vi "setup mfc LabJack interface.vi"() -> (0 "error out":errorcluster, 3 "LabJack Tasks":T2)   [LabVIEW 2021]
uses:
  temporal odor control/LabJack Interface/LabJackSetupChannel.ctl
  temporal odor control/LabJack Interface/LabJack AOAI Channel.ctl
panel:
  in  "Output Channels":T4={"OdorFlowRate"={"LabJack"=enum."1", "LabJack Channel Number"=0.0, "Scaling"=0.1}, "Background Air Flow"={"LabJack"=enum."1", "LabJack Channel Number"=1.0, "Scaling"=0.001}, "Air Dilution"={"LabJack"=enum."2", "LabJack Channel Number"=1.0, "Scaling"=0.025}}
  out "labjack2 handle":i32
  in  "Input Channels":T5={"OdorFlowRate"={"LabJack"=enum."1", "LabJack Channel Number"=2.0, "Scaling"=10.0}, "PID outlet"={"LabJack"=enum."1", "LabJack Channel Number"=0.0, "Scaling"=1.0}, "Outlet OpticalFlowSensor"={"LabJack"=enum."2", "LabJack Channel Number"=0.0, "Scaling"=1.0}, "Background Air Flow"={"LabJack"=enum."2", "LabJack Channel Number"=1.0, "Scaling"=1000.0}, "Air Dilution"={"LabJack"=enum."2", "LabJack Channel Number"=2.0, "Scaling"=40.0}}
  out "labjack1 handle":i32
  # "sccm/V"
  # "V/sccm"
  # "V/sccm"
  # "V/sccm"
  # "white = setpoint\nyellow = flow out\ngreen = valve off\nblue = purge"
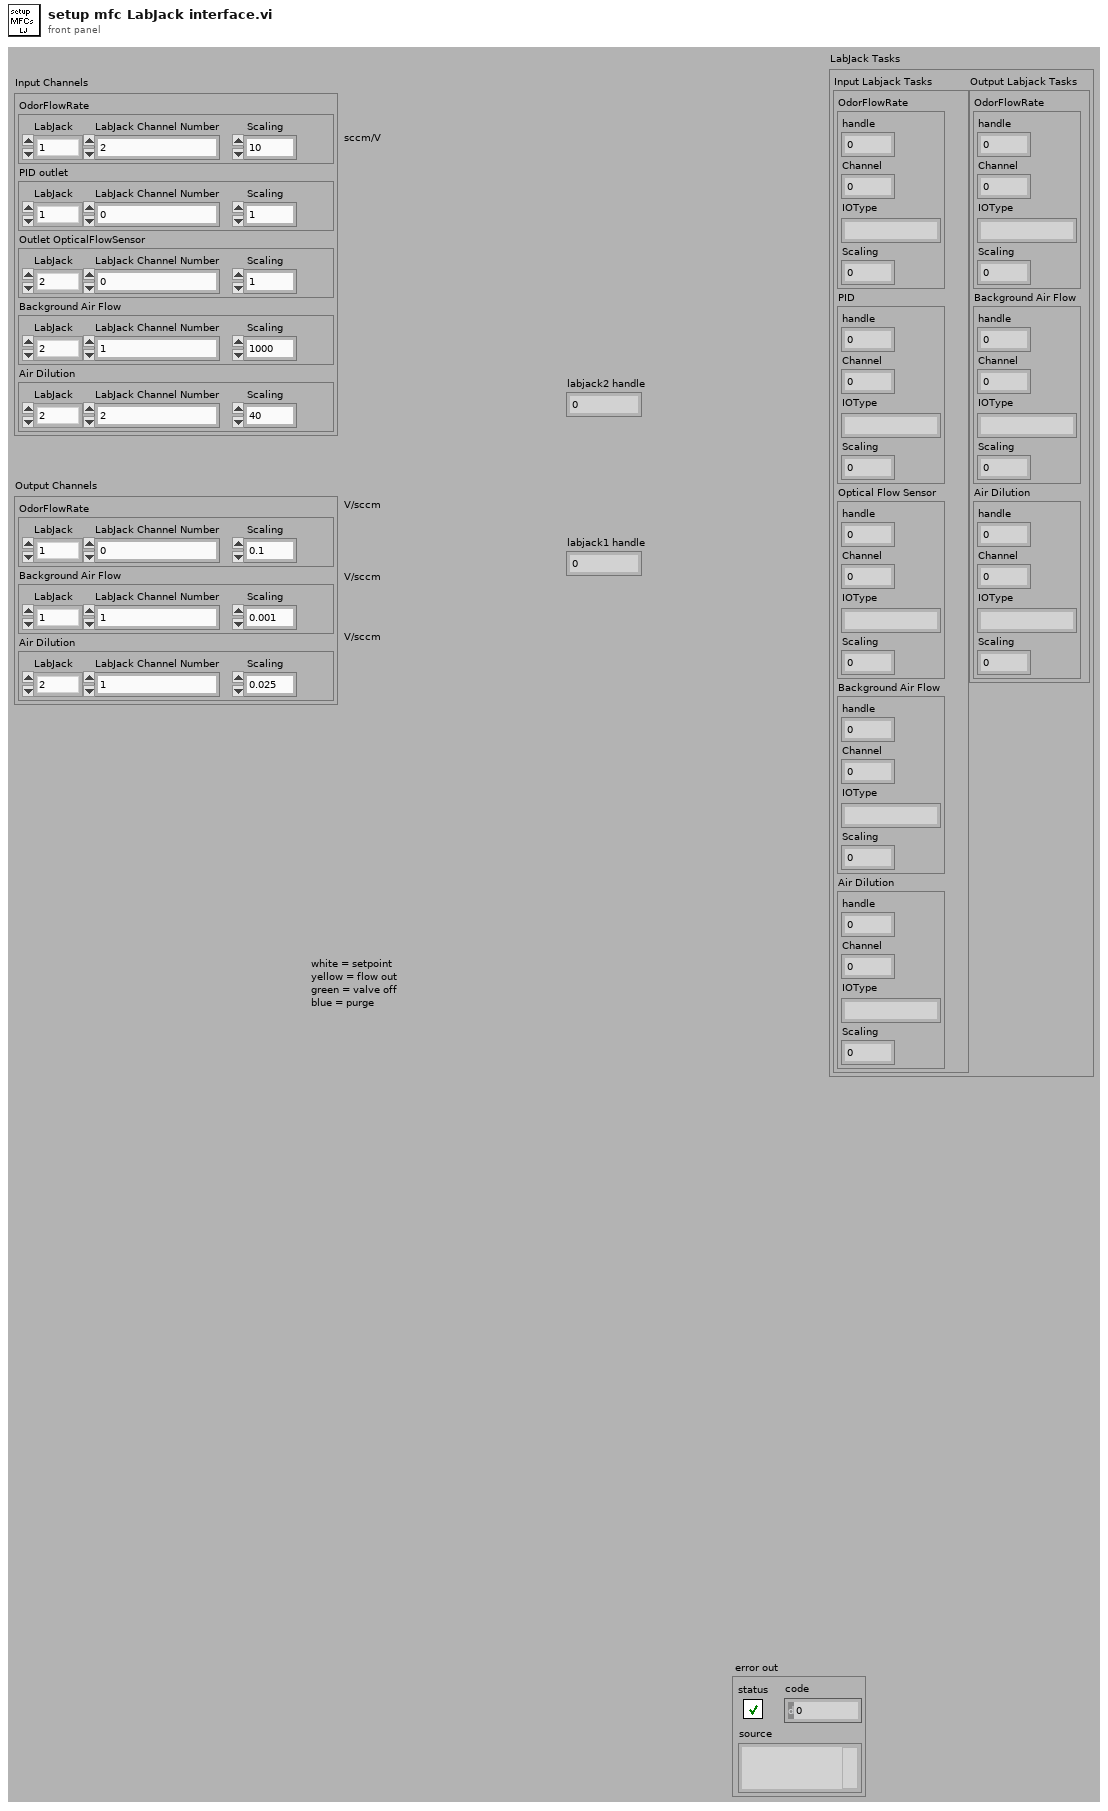
[diagram p1: front panel]
types:
  T1 = typedef "LabJack AOAI Channel.ctl" = cluster{"handle":i32, "Channel":i32, "IOType":string, "Scaling":dbl}
  T2 = cluster{"Input Labjack Tasks":cluster{"OdorFlowRate":T1, "PID":T1, "Optical Flow Sensor":T1, "Background Air Flow":T1, "Air Dilution":T1}, "Output Labjack Tasks":cluster{"OdorFlowRate":T1, "Background Air Flow":T1, "Air Dilution":T1}}
  T3 = typedef "LabJackSetupChannel.ctl" = cluster{"LabJack":enum16{"none", "1", "2", "1-FIO", "2-FIO"}, "LabJack Channel Number":dbl, "Scaling":dbl}
  T4 = cluster{"OdorFlowRate":T3, "Background Air Flow":T3, "Air Dilution":T3}
  T5 = cluster{"OdorFlowRate":T3, "PID outlet":T3, "Outlet OpticalFlowSensor":T3, "Background Air Flow":T3, "Air Dilution":T3}
  T6 = cluster{"[0]":T1, "[1]":T1, "[2]":T1, "[3]":T1, "[4]":T1}
  T7 = cluster{cluster{"[0]":T1, "[1]":T1, "[2]":T1, "[3]":T1, "[4]":T1}, cluster{"[0]":T1, "[1]":T1, "[2]":T1}}
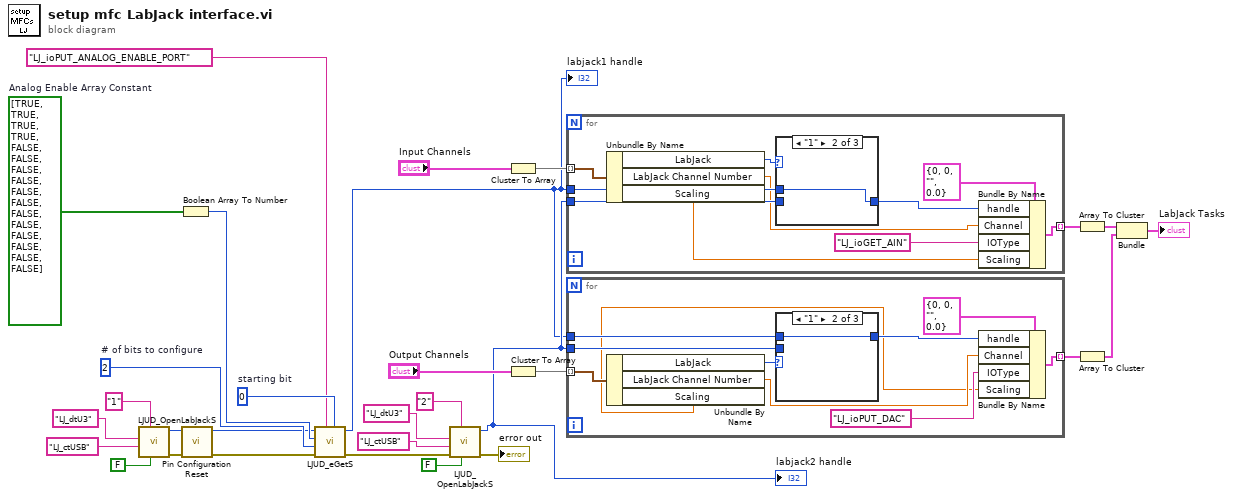
[diagram p0: block diagram]
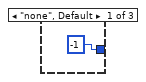
[diagram p2: hidden frame]
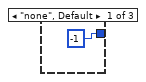
[diagram p4: hidden frame]
diagram:
  w21 = 2  # # of bits to configure
  w23 = 0  # starting bit
  w24 = bool[] [TRUE, TRUE, TRUE, TRUE, FALSE, FALSE, FALSE, FALSE, FALSE, FALSE, FALSE, FALSE, FALSE, FALSE, FALSE, FALSE]  # Analog Enable Array Constant
  n1 = call "LJUD_OpenLabJackS.vi"("FirstFound"=FALSE, "Address"="1" ("DeviceType"), "ConnectionType"="LJ_ctUSB", "DeviceType"="LJ_dtU3") -> ("error out"=w25:errorcluster, "Handle"=w26:i32)  [unwired: 5 in, 1 out]
  n2 = Boolean Array To Number(Boolean array=w24) -> (number=w20:u32)
  n3 = call "Pin Configuration Reset.vi"("error in"=w25, "Handle In"=w26) -> ("error out"=w18:errorcluster, "Handle Out"=w19:i32)  [unwired: 8 in]
  n4 = call "LJUD_eGetS.vi"("Channel"=w23, "IOType"="LJ_ioPUT_ANALOG_ENABLE_PORT", "error in"=w18, "x1"=w21, "Value Write"=w20, "Handle In"=w19) -> ("error out"=w5:errorcluster, "Handle Out"=w6:i32)  [unwired: 3 in, 1 out]
  "labjack1 handle" <- w6
  n5 = call "LJUD_OpenLabJackS.vi"("FirstFound"=FALSE, "Address"="2", "error in"=w5, "ConnectionType"="LJ_ctUSB", "DeviceType"="LJ_dtU3") -> ("error out"=→"error out":errorcluster, "Handle"=w7:i32)  [unwired: 4 in, 1 out]
  "labjack2 handle" <- w7
  n6 = Cluster To Array(cluster="Input Channels") -> (array=w10:T3[])
  n7 = Cluster To Array(cluster="Output Channels") -> (array=w12:T3[])
  n8 = for {
    tunnel: w6 -> [w38]
    tunnel: w10 -> [w40] mode=indexing
    tunnel: w7 -> [w37]
    tunnel: [w33] -> w9 mode=indexing
    n9 = Unbundle By Name(w40) -> ("LabJack"=w39:enum16{"none", "1", "2", "1-FIO", "2-FIO"}, "LabJack Channel Number"=w34:dbl, "Scaling"=w31:dbl)
    n10 = case shown="\"1\"" w39 {
      tunnel: w38 -> [_ w42 _]
      tunnel: w37 -> [_ _ w43]
      tunnel: [-1 ("Handle") w42 w43] -> w35
      frame "none", Default {
      }
      frame "1" {
      }
      frame "2" {
      }
    }
    n11 = Bundle By Name(cluster=T1 {"handle"=0, "Channel"=0, "IOType"="", "Scaling"=0.0} ("LabJack AO/AI Channel"), "handle"=w35, "Channel"=w34, "IOType"="LJ_ioGET_AIN", "Scaling"=w31) -> (w33:T1)
  }
  n12 = for {
    tunnel: w6 -> [w51]
    tunnel: w12 -> [w53] mode=indexing
    tunnel: w7 -> [w50]
    tunnel: [w45] -> w11 mode=indexing
    n13 = Unbundle By Name(w53) -> ("LabJack"=w52:enum16{"none", "1", "2", "1-FIO", "2-FIO"}, "LabJack Channel Number"=w47:dbl, "Scaling"=w44:dbl)
    n14 = case shown="\"1\"" w52 {
      tunnel: w51 -> [_ w55 _]
      tunnel: w50 -> [_ _ w56]
      tunnel: [-1 ("Handle") w55 w56] -> w48
      frame "none", Default {
      }
      frame "1" {
      }
      frame "2" {
      }
    }
    n15 = Bundle By Name(cluster=T1 {"handle"=0, "Channel"=0, "IOType"="", "Scaling"=0.0} ("LabJack AO/AI Channel"), "handle"=w48, "Channel"=w47, "IOType"="LJ_ioPUT_DAC", "Scaling"=w44) -> (w45:T1)
  }
  n16 = Array To Cluster(array=w9) -> (cluster=w3:T6)
  n17 = Array To Cluster(array=w11) -> (cluster=w2:cluster{"[0]":T1, "[1]":T1, "[2]":T1})
  n18 = Bundle(w3, w2) -> (→"LabJack Tasks":T7)  [unwired: 1 in]
